vi "GetRightClickMenu.vi"(0 "reference":refnum<class "StateDiagramGraph.lvclass">, 5 "error in (no error)":errorcluster) -> (14 "reference out":refnum<class "StateDiagramGraph.lvclass">, 15 "Array":string[](array[string]), 16 "Found":bool, 19 "error out":errorcluster)   [LabVIEW 2012, in "StateDiagramGraph.lvclass"]
doc: "GetRightClickMenu"
uses:
  <resource>/Framework/Providers/Open_GDS/UML/StateDiagramGraph_class/StateDiagramGraph.lvclass
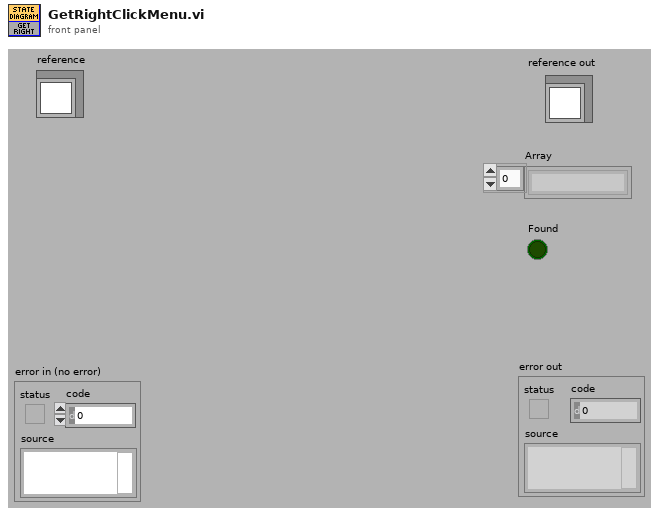
[diagram p1: front panel]
types:
  T1 = typedef "StateDiagramGraph.lvclass/ObjectAttributes.ctl" = cluster{"Base class":T2, "StateDiagramData":T3}
  T2 = typedef "Graph.lvclass/ObjectAttributes.ctl" = cluster{"nodes":refnum<class "AbstractNode.lvclass">[], "edges":refnum<class "AbstractEdge.lvclass">[], "nodesToBeRemoved":refnum<class "AbstractNode.lvclass">[], "edgesToBeRemoved":refnum<class "AbstractEdge.lvclass">[], "needsLayout":bool, "LayoutNodes":refnum<class "AbstractNode.lvclass">[]}
  T3 = typedef "StateDiagramGraph.lvclass/StateDiagramData.ctl" = cluster{"VI-Path":path, "ShowOption":T4}
  T4 = typedef "StateDiagramGraph.lvclass/ViPathShowOption.ctl" = enum16{"Don't Show", "Show Relative Path", "Show Absolute Path"}
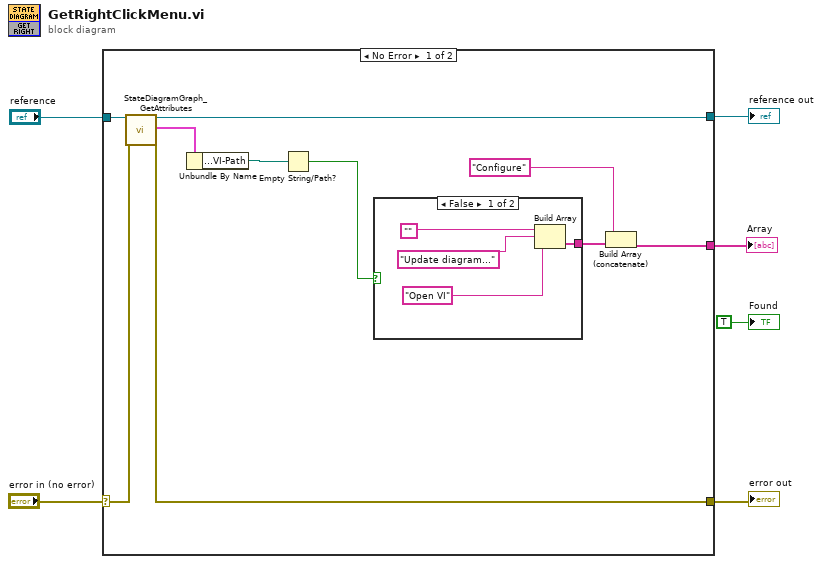
[diagram p0: block diagram]
diagram:
  n1 = case shown="No Error" "error in (no error)" {
    selector: "error in (no error)" -> [w16 w21]
    tunnel: "reference" -> [w15 w22]
    tunnel: [w12 w21] -> w4
    tunnel: [w13 w22] -> w3
    tunnel: [w10 _] -> w2
    frame No Error {
      n2 = call <resource>:"StateDiagramGraph_GetAttributes.vi"("reference in"=w15, "error in (no error)"=w16) -> ("reference out"=w13:refnum<class "StateDiagramGraph.lvclass">, "Attributes"=w14:T1, "error out"=w12:errorcluster)  [unwired: 15 out]
      n3 = Unbundle By Name(w14) -> ("StateDiagramData.VI-Path"=w11:path)
      n4 = Empty String/Path?(string/path=w11) -> (empty?=w9:bool)
      n5 = case shown="False" w9 {
        tunnel: [w18 _] -> w7
        frame False {
          n6 = Build Array("", "Update diagram...", "Open VI") -> (w18:string[])
        }
        frame True {
        }
      }
      n7 = Build Array (concatenate)("Configure", w7) -> (w10:string[])
    }
    frame Error {
    }
  }
  "reference out" <- w3
  "error out" <- w4
  "Array" <- w2
  "Found" <- TRUE ("Found")
